vi "Search ID by Name.vi"(8 "error in (no error)":errorcluster, 9 "ID":string, 10 "Hue Config":T1) -> (0 "error out":errorcluster, 2 "ID":u8)   [LabVIEW 2020, in "LMH-Hue.lvlib"]
uses:
  LMH-Hue.lvlib
  Type Defs/Hue Ref.ctl
  <vilib>/httpClient/ClientHandle.ctl
  Type Defs/Light Data.ctl
  3d9aac69-2a40-4ca4-b0c0-ef428fe3223d.vi
  <vilib>/httpClient/LabVIEWHTTPClient.lvlib
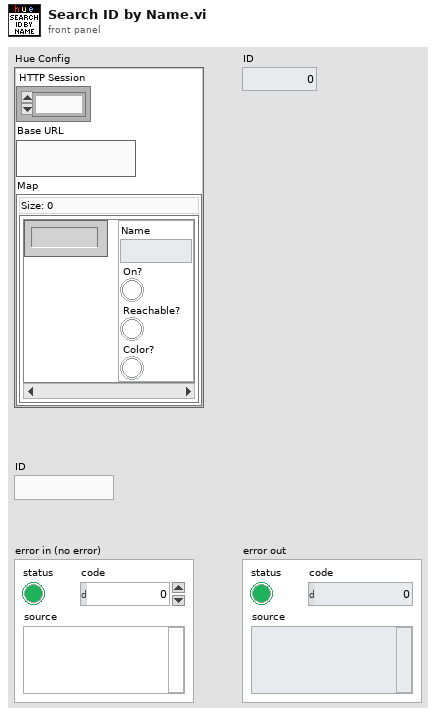
[diagram p1: front panel]
types:
  T1 = typedef "LMH-Hue.lvlib/Hue Ref.ctl" = cluster{"HTTP Session":T2, "Base URL":string, "Map":map{i32, T3}}
  T2 = typedef "LabVIEWHTTPClient.lvlib/ClientHandle.ctl" = refnum<k1>
  T3 = typedef "LMH-Hue.lvlib/Light Data.ctl" = cluster{"Name":string, "On?":bool, "Reachable?":bool, "Color?":bool}
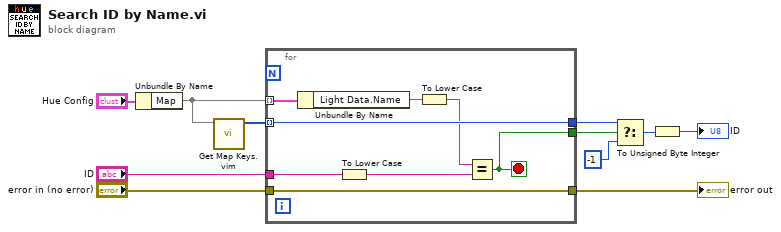
[diagram p0: block diagram]
diagram:
  n1 = Unbundle By Name("Hue Config") -> ("Map"=w2:map{i32, T3})
  n2 = call "Get Map Keys.vim"("Map"=w2) -> ("Key Array"=w1:i32[])  [unwired: 10 in]
  n3 = for {
    tunnel: w2 -> [w19] mode=indexing
    tunnel: w1 -> [w16] mode=indexing
    tunnel: "ID" -> [w18]
    tunnel: "error in (no error)" -> [w15]
    tunnel: [w16] -> w9
    tunnel: [w15] -> w5
    tunnel: [w12] -> w6
    stop <- w12 stop-if-true
    n4 = Unbundle By Name(w19) -> ("Light Data.Name"=w17:string)
    n5 = To Lower Case(string=w18) -> (all lower case string=w14:string)
    n6 = To Lower Case(string=w17) -> (all lower case string=w13:string)
    n7 = Equal?(x=w13, y=w14) -> (x = y?=w12:bool)
  }
  "error out" <- w5
  n8 = Select(t=w9, s=w6, f=-1) -> (s? t:f=w8:i32)
  n9 = To Unsigned Byte Integer(number=w8) -> (unsigned 8bit integer=→"ID":u8)
